vi "Auto_Shooting.vi"(8 "Tip Bridge in auto":bool=TRUE, 10 "Previous Outputs":T8, 11 "Sensor Inputs":T1) -> (0 "Roller Commands":T23, 1 "Tipper Command Inputs":T22, 2 "Turret Command Inputs":T19, 3 "Conveyor Command Inputs":T20, 4 "Flywheel Commands":T24, 5 "Drive Command Inputs":T21)   [LabVIEW 2012]
uses:
  Flywheel/Input_Commands_Flywheel.ctl
  Roller/Input_Commands_Roller.ctl
  Bridge Tipper/Inputs_Tipper.ctl
  tankdrive/Input_Commands_Drive.ctl
  Conveyor/Input_Command_Conveyor.ctl
  Turret/Inputs_Commands_Turret.ctl
  Outputs_All.ctl
  Flywheel/Outputs_Flywheel.ctl
  tankdrive/Output_Wheel_Speeds.ctl
  Conveyor/Conveyor_outputs.ctl
  Conveyor/Conveyor module state.ctl
  Conveyor/Conveyor_outputsV2.ctl
  Conveyor/3-Ball-Conveyor_Module_State.ctl
  Conveyor/T_Roller module state.ctl
  Turret/Outputs_Turret.ctl
  Roller/Outputs_Roller.ctl
  Bridge Tipper/Outputs_Tipper.ctl
  Inputs_All.ctl
  Flywheel/Sensor_Inputs_FlyWheel.ctl
  tankdrive/Input_Sensors_Drive.ctl
  Conveyor/Sensor_Input_Conveyor.ctl
  Conveyor/Sensor_Input_ConveyorV2.ctl
  Turret/Inputs_Sensors_Turret.ctl
  Inputs_Camera.ctl
  Autonomous Shooting State.ctl
panel:
  in  "Wait time":u32=1500
  in  "Approach time":u32=700
  in  "Bridge tipping time":u32=4000
  in  "Shoot time":u32=4000
  in  "Wheel spin up time":u32=4000
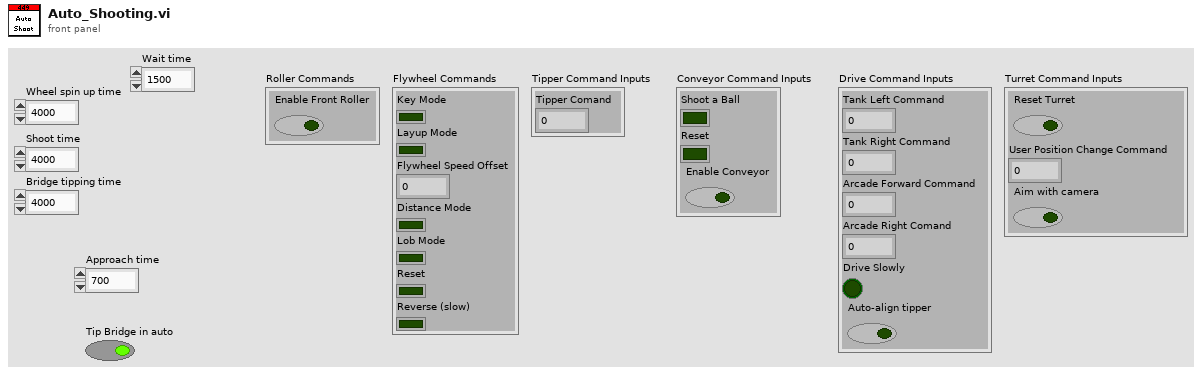
[diagram p1: front panel]
types:
  T1 = typedef "Inputs_All.ctl" = cluster{"Inputs_FlyWheel":T2, "Drive Inputs":T3, "Conveyor Inputs":T4, "ConveyorV2 Inputs":T5, "Turret Inputs":T6, "Camera Inputs":T7}
  T2 = typedef "Sensor_Inputs_FlyWheel.ctl" = cluster{"Speed":dbl, "Target Distance":dbl}
  T3 = typedef "Input_Sensors_Drive.ctl" = cluster{"Left Front Speed":dbl, "Right Front Speed":dbl, "Left Back Speed":dbl, "Right Back Speed":dbl}
  T4 = typedef "Sensor_Input_Conveyor.ctl" = cluster{"Top Ball Detector Count":i32, "Bottom Ball Detector Count":i32, "Shooter Ball Detector Count":i32}
  T5 = typedef "Sensor_Input_ConveyorV2.ctl" = cluster{"Grab Ball Detector Count":i32, "Bottom Ball Detector Count":i32, "Top In Place Ball Detector Count":i32, "Top Too Far Ball Detector Count":i32, "Top Not Far Enough":i32}
  T6 = typedef "Inputs_Sensors_Turret.ctl" = cluster{"At Minimum Angle":bool, "At Maximum Angle":bool, "Camera Position Offset":dbl, "Found Target?":bool, "Position Encoder":dbl}
  T7 = typedef "Inputs_Camera.ctl" = cluster{"Offset Angle from Perpendicular (degrees)":dbl, "Target Dist":dbl, "Elevation Angle":dbl, "Found Target":bool, "Bounding Rect":cluster{"Left":dbl, "Top":dbl, "Right":dbl, "Bottom":dbl}}
  T8 = typedef "Outputs_All.ctl" = cluster{"Flywheel Outputs":T9, "Drive Outputs":T10, "Conveyor Outputs":T11, "Conveyor Outputs 2":T13, "Turret Outputs":T16, "Roller Outputs":T17, "Bridge Tipper Outputs":T18}
  T9 = typedef "Outputs_Flywheel.ctl" = cluster{"Wheel Speed":dbl}
  T10 = typedef "Output_Wheel_Speeds.ctl" = cluster{"Front Left Speed":dbl, "Front Right Speed":dbl, "Back Left Speed":dbl, "Back Right Speed":dbl}
  T11 = typedef "Conveyor_outputs.ctl" = cluster{"Bottom Conveyor Speed":dbl, "Top Conveyor Speed":dbl, "Bottom Conveyor State":T12, "Top Conveyor State":T12, "Accepting Balls":bool, "Number of Balls":i32}
  T12 = typedef "Conveyor module state.ctl" = enum16{"No Ball", "Has Ball", "Ball Below Hold", "Ball Above Hold", "Outputting Ball", "Reset"}
  T13 = typedef "Conveyor_outputsV2.ctl" = cluster{"Accepting Balls":bool, "Number of Balls":i32, "Conveyor State":T14, "Top Roller State":T15, "Top Roller":dbl, "Conveyor":dbl}
  T14 = typedef "3-Ball-Conveyor_Module_State.ctl" = enum16{"No Balls", "Collecting Ball", "Holding 1", "Pushing Ball Out", "Holding 2", "Lowering Ball", "Reset", "Disabled"}
  T15 = typedef "T_Roller module state.ctl" = enum16{"Reset", "Disabled", "Waiting for Ball", "Holding", "Ball not far enough", "Ball too far", "Firing"}
  T16 = typedef "Outputs_Turret.ctl" = cluster{"Desired Position":dbl, "Is Reset":bool, "Target In Deadzone":bool}
  T17 = typedef "Outputs_Roller.ctl" = cluster{"Front Roller":dbl}
  T18 = typedef "Outputs_Tipper.ctl" = cluster{"Speed":dbl}
  T19 = typedef "Inputs_Commands_Turret.ctl" = cluster{"Reset Turret":bool, "User Position Change Command":dbl, "Aim with camera":bool}
  T20 = typedef "Input_Command_Conveyor.ctl" = cluster{"Shoot a Ball":bool, "Reset":bool, "Enable Conveyor":bool}
  T21 = typedef "Input_Commands_Drive.ctl" = cluster{"Tank Left Command":dbl, "Tank Right Command":dbl, "Arcade Forward Command":dbl, "Arcade Right Comand":dbl, "Drive Slowly":bool, "Auto-align tipper":bool}
  T22 = typedef "Inputs_Tipper.ctl" = cluster{"Tipper Comand":dbl}
  T23 = typedef "Input_Commands_Roller.ctl" = cluster{"Enable Front Roller":bool}
  T24 = typedef "Input_Commands_Flywheel.ctl" = cluster{"Key Mode":bool, "Layup Mode":bool, "Flywheel Speed Offset":dbl, "Distance Mode":bool, "Lob Mode":bool, "Reset":bool, "Reverse (slow)":bool}
  T25 = typedef "Autonomous Shooting State.ctl" = enum16{"Approach Target", "Wait", "Spin up flywheel", "Shooting", "Hit bridge", "Done"}
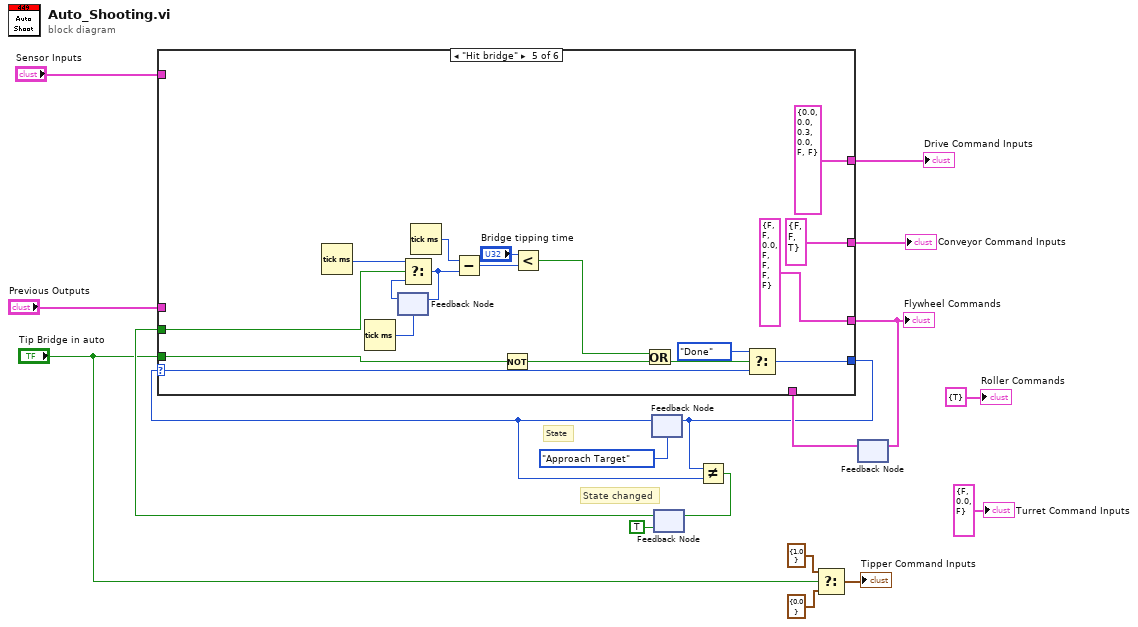
[diagram p0: block diagram]
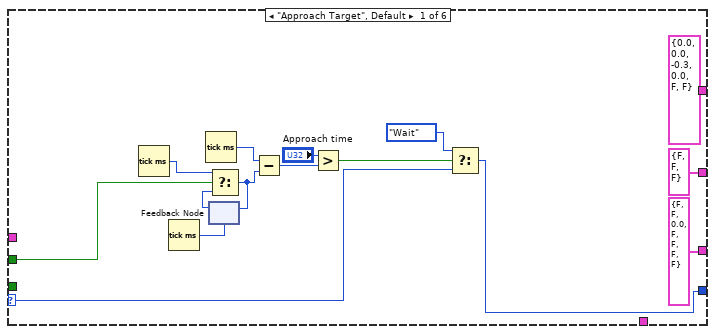
[diagram p2: hidden frame]
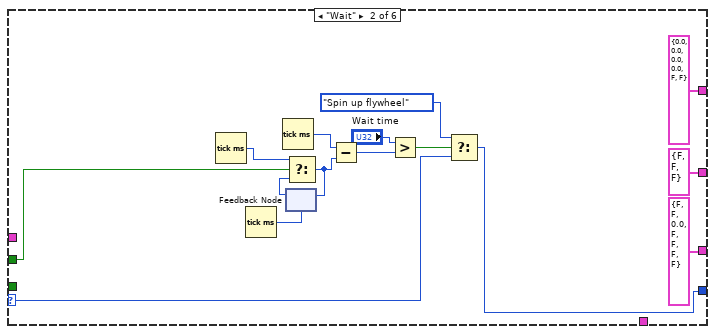
[diagram p3: hidden frame]
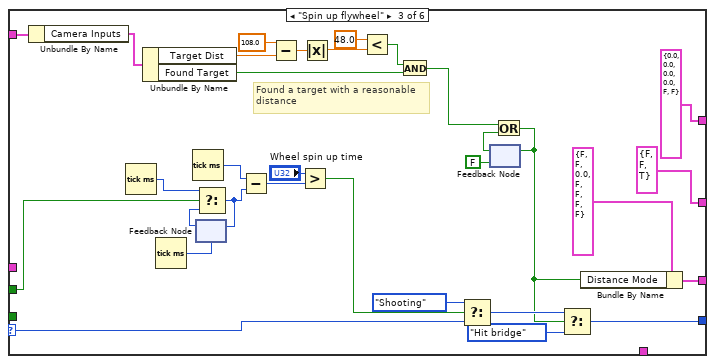
[diagram p4: hidden frame]
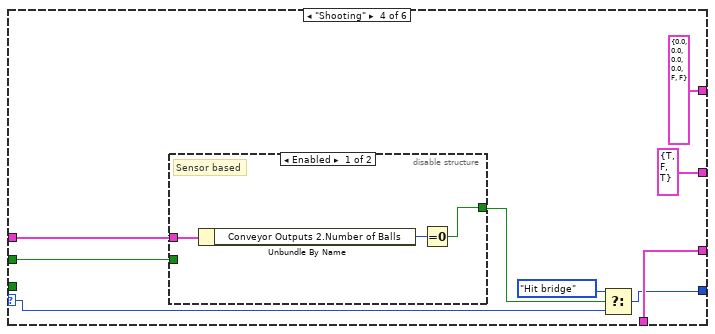
[diagram p5: hidden frame]
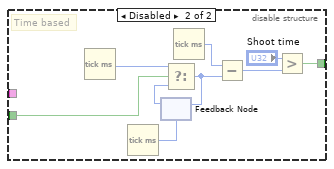
[diagram p6: hidden frame]
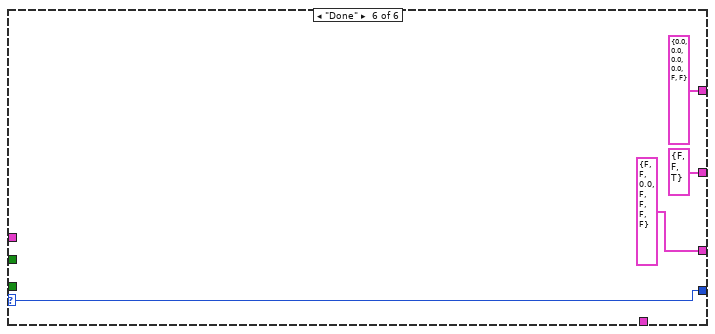
[diagram p7: hidden frame]
diagram:
  # "State changed"
  # "State"
  n1 = feedback #1(Autonomous_Shooting_State."Approach Target" ("Auto States")) -> (w15:T25)
  n2 = feedback #2(TRUE) -> (w12:bool)
  n3 = Select(t=T22 {"Tipper Comand"=1.0} ("Tipper Command Inputs"), s="Tip Bridge in auto", f=T22 {"Tipper Comand"=0.0} ("Tipper Command Inputs")) -> (s? t:f=→"Tipper Command Inputs":T22)
  n4 = feedback #3() -> (w10:T24)  [unwired: 1 in]
  n5 = case shown="\"Hit bridge\"" w15 {
    selector: w15 -> [w21 w36 w56 w84 w107 w122]
    tunnel: [T24 {"Key Mode"=FALSE, "Layup Mode"=FALSE, "Flywheel Speed Offset"=0.0, "Distance Mode"=FALSE, "Lob Mode"=FALSE, "Reset"=FALSE, "Reverse (slow)"=FALSE} ("Flywheel Commands") T24 {"Key Mode"=FALSE, "Layup Mode"=FALSE, "Flywheel Speed Offset"=0.0, "Distance Mode"=FALSE, "Lob Mode"=FALSE, "Reset"=FALSE, "Reverse (slow)"=FALSE} ("Flywheel Commands") w78 w88 T24 {"Key Mode"=FALSE, "Layup Mode"=FALSE, "Flywheel Speed Offset"=0.0, "Distance Mode"=FALSE, "Lob Mode"=FALSE, "Reset"=FALSE, "Reverse (slow)"=FALSE} ("Flywheel Commands") T24 {"Key Mode"=FALSE, "Layup Mode"=FALSE, "Flywheel Speed Offset"=0.0, "Distance Mode"=FALSE, "Lob Mode"=FALSE, "Reset"=FALSE, "Reverse (slow)"=FALSE} ("Flywheel Commands")] -> w11
    tunnel: "Sensor Inputs" -> [_ _ w77 _ _ _]
    tunnel: w12 -> [w26 w38 w63 w85 w110 _]
    tunnel: [w19 w34 w50 w81 w105 w122] -> w5
    tunnel: w10 -> [_ _ _ w88 _ _]
    tunnel: [T20 {"Shoot a Ball"=FALSE, "Reset"=FALSE, "Enable Conveyor"=FALSE} ("Conveyor Command Inputs") T20 {"Shoot a Ball"=FALSE, "Reset"=FALSE, "Enable Conveyor"=FALSE} ("Conveyor Command Inputs") T20 {"Shoot a Ball"=FALSE, "Reset"=FALSE, "Enable Conveyor"=TRUE} ("Conveyor Command Inputs") T20 {"Shoot a Ball"=TRUE, "Reset"=FALSE, "Enable Conveyor"=TRUE} ("Conveyor Command Inputs") T20 {"Shoot a Ball"=FALSE, "Reset"=FALSE, "Enable Conveyor"=TRUE} ("Conveyor Command Inputs") T20 {"Shoot a Ball"=FALSE, "Reset"=FALSE, "Enable Conveyor"=TRUE} ("Conveyor Command Inputs")] -> w9
    tunnel: "Previous Outputs" -> [_ _ _ w86 _ _]
    tunnel: [T21 {"Tank Left Command"=0.0, "Tank Right Command"=0.0, "Arcade Forward Command"=-0.3, "Arcade Right Comand"=0.0, "Drive Slowly"=FALSE, "Auto-align tipper"=FALSE} ("Drive Command Inputs") T21 {"Tank Left Command"=0.0, "Tank Right Command"=0.0, "Arcade Forward Command"=0.0, "Arcade Right Comand"=0.0, "Drive Slowly"=FALSE, "Auto-align tipper"=FALSE} ("Drive Command Inputs") T21 {"Tank Left Command"=0.0, "Tank Right Command"=0.0, "Arcade Forward Command"=0.0, "Arcade Right Comand"=0.0, "Drive Slowly"=FALSE, "Auto-align tipper"=FALSE} ("Drive Command Inputs") T21 {"Tank Left Command"=0.0, "Tank Right Command"=0.0, "Arcade Forward Command"=0.0, "Arcade Right Comand"=0.0, "Drive Slowly"=FALSE, "Auto-align tipper"=FALSE} ("Drive Command Inputs") T21 {"Tank Left Command"=0.0, "Tank Right Command"=0.0, "Arcade Forward Command"=0.3, "Arcade Right Comand"=0.0, "Drive Slowly"=FALSE, "Auto-align tipper"=FALSE} ("Drive Command Inputs") T21 {"Tank Left Command"=0.0, "Tank Right Command"=0.0, "Arcade Forward Command"=0.0, "Arcade Right Comand"=0.0, "Drive Slowly"=FALSE, "Auto-align tipper"=FALSE} ("Drive Command Inputs")] -> w6
    tunnel: "Tip Bridge in auto" -> [_ _ _ _ w102 _]
    frame "Approach Target", Default {
      n6 = Tick Count (ms)() -> (millisecond timer value=w31:u32)
      n7 = Tick Count (ms)() -> (millisecond timer value=w33:u32)
      n8 = Tick Count (ms)() -> (millisecond timer value=w30:u32)
      n9 = feedback #4(w33) -> (w32:u32)
      n10 = Select(t=w31, s=w26, f=w32) -> (s? t:f=w29:u32)
      n11 = feedback-in #4(w29) -> ()
      n12 = Subtract(x=w30, y=w29) -> (x-y=w28:u32)
      n13 = Greater?(x="Approach time", y=w28) -> (0:w22:bool)
      n14 = Select(t=Autonomous_Shooting_State."Wait", s=w22, f=w21) -> (s? t:f=w19:T25)
    }
    frame "Wait" {
      n15 = Tick Count (ms)() -> (millisecond timer value=w43:u32)
      n16 = Tick Count (ms)() -> (millisecond timer value=w45:u32)
      n17 = Tick Count (ms)() -> (millisecond timer value=w42:u32)
      n18 = feedback #5(w45) -> (w44:u32)
      n19 = Select(t=w43, s=w38, f=w44) -> (s? t:f=w41:u32)
      n20 = feedback-in #5(w41) -> ()
      n21 = Subtract(x=w42, y=w41) -> (x-y=w40:u32)
      n22 = Greater?(x="Wait time", y=w40) -> (0:w37:bool)
      n23 = Select(t=Autonomous_Shooting_State."Spin up flywheel", s=w37, f=w36) -> (s? t:f=w34:T25)
    }
    frame "Spin up flywheel" {
      # "Found a target with a reasonable\ndistance"
      n24 = Unbundle By Name(w77) -> ("Camera Inputs"=w76:T7)
      n25 = Tick Count (ms)() -> (millisecond timer value=w62:u32)
      n26 = Unbundle By Name(w76) -> ("Target Dist"=w73:dbl, "Found Target"=w67:bool)
      n27 = Tick Count (ms)() -> (millisecond timer value=w65:u32)
      n28 = Tick Count (ms)() -> (millisecond timer value=w61:u32)
      n29 = feedback #6(w65) -> (w64:u32)
      n30 = Select(t=w62, s=w63, f=w64) -> (s? t:f=w60:u32)
      n31 = feedback-in #6(w60) -> ()
      n32 = Subtract(x=w61, y=w60) -> (x-y=w59:u32)
      n33 = Subtract(x=108.0, y=w73) -> (x-y=w71:dbl)
      n34 = Greater?(x="Wheel spin up time", y=w59) -> (0:w57:bool)
      n35 = Absolute Value(x=w71) -> (abs(x)=w70:dbl)
      n36 = Less?(x=48.0, y=w70) -> (x < y?=w68:bool)
      n37 = And(x=w68, y=w67) -> (x .and. y?=w66:bool)
      n38 = Select(t=Autonomous_Shooting_State."Shooting", s=w57, f=w56) -> (s? t:f=w52:T25)
      n39 = feedback #7(FALSE) -> (w75:bool)
      n40 = Or(x=w66, y=w75) -> (x .or. y?=w51:bool)
      n41 = feedback-in #7(w51) -> ()
      n42 = Select(t=w52, s=w51, f=Autonomous_Shooting_State."Hit bridge") -> (s? t:f=w50:T25)
      n43 = Bundle By Name(cluster=T24 {"Key Mode"=FALSE, "Layup Mode"=FALSE, "Flywheel Speed Offset"=0.0, "Distance Mode"=FALSE, "Lob Mode"=FALSE, "Reset"=FALSE, "Reverse (slow)"=FALSE} ("Flywheel Commands"), "Distance Mode"=w51) -> (w78:T24)
    }
    frame "Shooting" {
      n44 = disable-structure shown="Enabled" {
        disable-tunnel: w86 -> [w91 _]
        disable-tunnel: [w89 w92] -> w83
        disable-tunnel: w85 -> [_ w98]
        frame Enabled {
          # "Sensor based"
          n45 = Unbundle By Name(w91) -> ("Conveyor Outputs 2.Number of Balls"=w90:i32)
          n46 = Equal To 0?(x=w90) -> (x = 0?=w89:bool)
        }
        frame Disabled {
          # "Time based"
          n47 = Tick Count (ms)() -> (millisecond timer value=w100:u32)
          n48 = Tick Count (ms)() -> (millisecond timer value=w97:u32)
          n49 = feedback #8(w97) -> (w99:u32)
          n50 = Select(t=w100, s=w98, f=w99) -> (s? t:f=w95:u32)
          n51 = feedback-in #8(w95) -> ()
          n52 = Tick Count (ms)() -> (millisecond timer value=w96:u32)
          n53 = Subtract(x=w96, y=w95) -> (x-y=w94:u32)
          n54 = Greater?(x="Shoot time", y=w94) -> (0:w92:bool)
        }
      }
      n55 = Select(t=Autonomous_Shooting_State."Hit bridge", s=w83, f=w84) -> (s? t:f=w81:T25)
    }
    frame "Hit bridge" {
      n56 = Tick Count (ms)() -> (millisecond timer value=w111:u32)
      n57 = Tick Count (ms)() -> (millisecond timer value=w113:u32)
      n58 = feedback #9(w113) -> (w112:u32)
      n59 = Select(t=w111, s=w110, f=w112) -> (s? t:f=w115:u32)
      n60 = feedback-in #9(w115) -> ()
      n61 = Tick Count (ms)() -> (millisecond timer value=w114:u32)
      n62 = Subtract(x=w114, y=w115) -> (x-y=w109:u32)
      n63 = Not(x=w102) -> (.not. x?=w101:bool)
      n64 = Less?(x="Bridge tipping time", y=w109) -> (x < y?=w103:bool)
      n65 = Or(x=w103, y=w101) -> (x .or. y?=w104:bool)
      n66 = Select(t=Autonomous_Shooting_State."Done", s=w104, f=w107) -> (s? t:f=w105:T25)
    }
    frame "Done" {
    }
  }
  "Flywheel Commands" <- w11
  "Drive Command Inputs" <- w6
  "Conveyor Command Inputs" <- w9
  n67 = feedback-in #1(w5) -> ()
  n68 = Not Equal?(x=w5, y=w15) -> (x != y?=w14:bool)
  n69 = feedback-in #2(w14) -> ()
  n70 = feedback-in #3(w11) -> ()
  "Roller Commands" <- T23 {"Enable Front Roller"=TRUE} ("Roller Commands")
  "Turret Command Inputs" <- T19 {"Reset Turret"=FALSE, "User Position Change Command"=0.0, "Aim with camera"=FALSE} ("Turret Command Inputs")
